vi "Scanner - Top VI.vi"(8 "error in":errorcluster) -> (0 "error out":errorcluster)   [LabVIEW 2024, in "Session Scanner.lvlib"]
uses:
  Session Scanner.lvlib
  Scanner Queue - Dequeue.vi
  User Interface/UI Queue - Enqueue.vi
  Scanner Queue - Enqueue.vi
  Support/General Type Defs/Global Data.vi
  Scanner Queue - Destroy.vi
  User Interface/User Interface.lvlib
  Support/General Type Defs/General Type Defs.lvlib
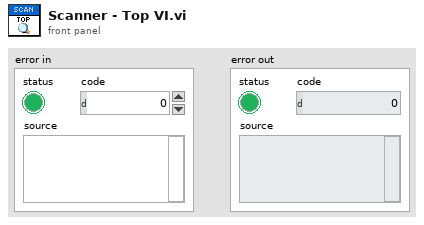
[diagram p1: front panel]
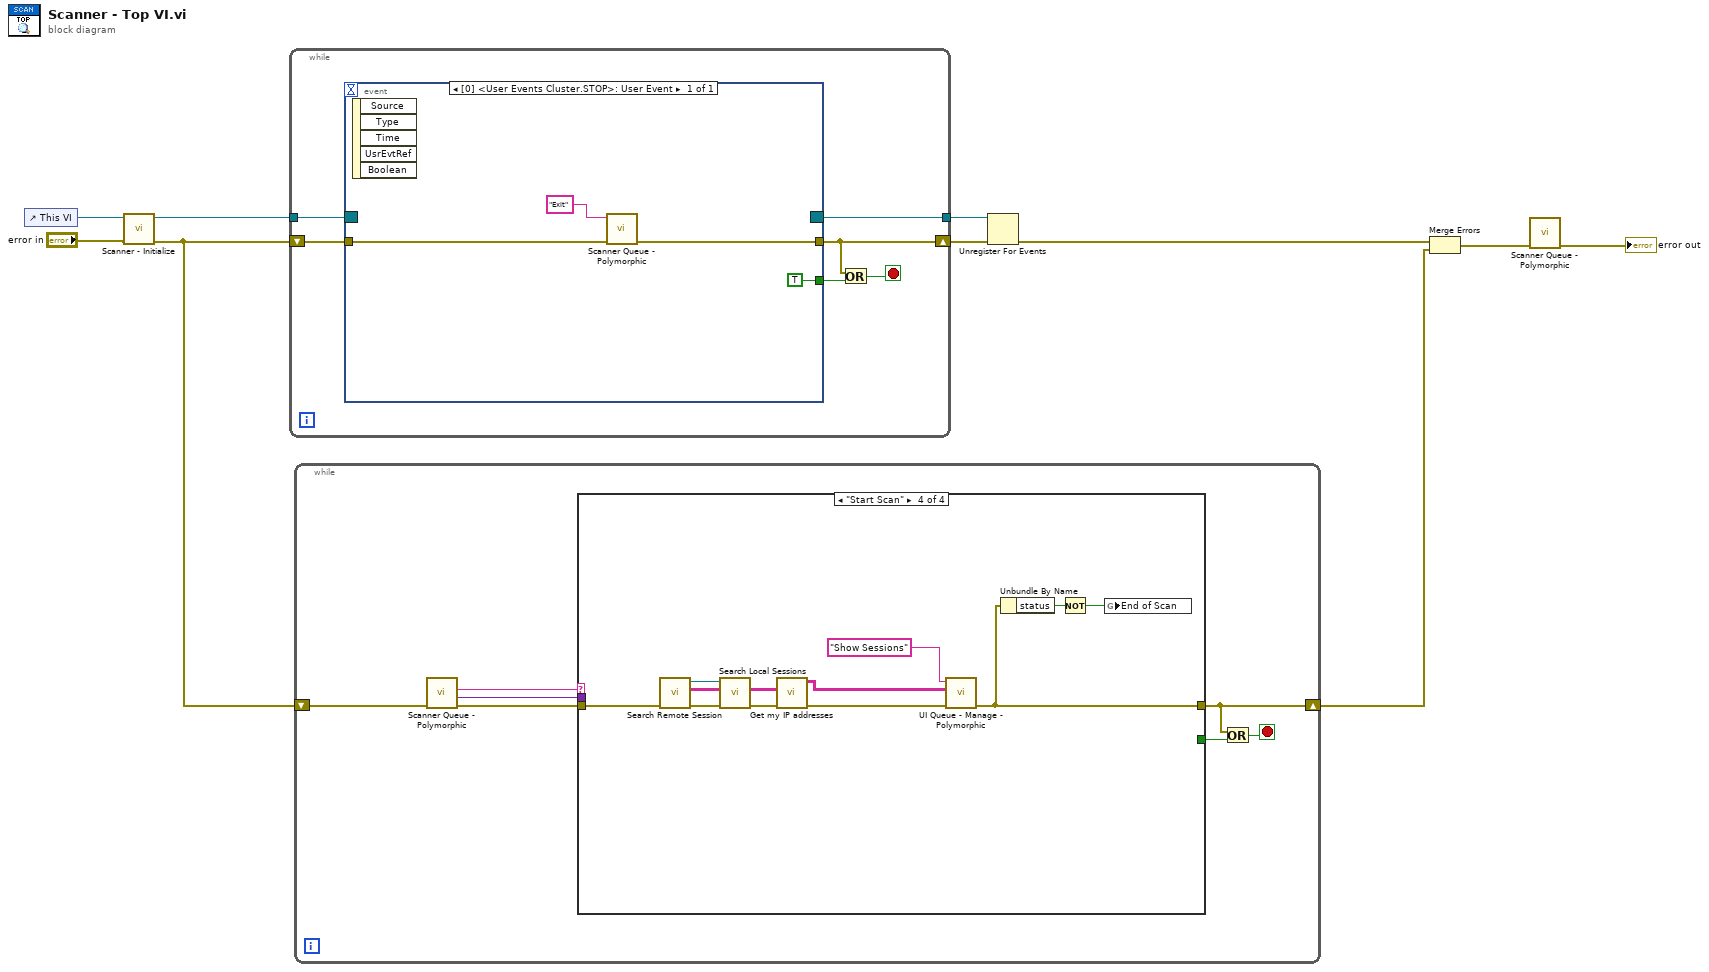
[diagram p0: block diagram]
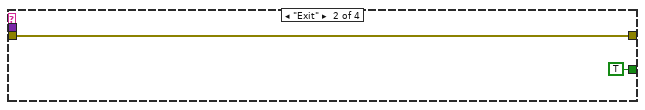
[diagram p3: hidden frame]
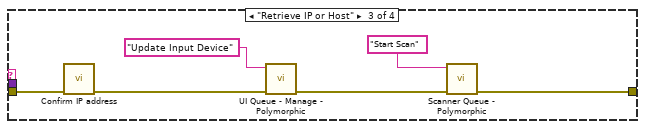
[diagram p4: hidden frame]
diagram:
  n1 = control-ref of="This VI"() -> (w1:refnum<vi>)
  n2 = call "Scanner - Initialize.vi"("error in (no error)"="error in", "VI In"=w1) -> ("error out"=w6:errorcluster, "Event Registration Out"=w9:refnum<event-registration>)  [unwired: 8 in]
  n3 = while {
    tunnel: w9 -> [w16]
    shift-right: [w11] -> w8
    shift-left: w6 -> [w15]
    tunnel: [w14] -> w7
    stop <- w12 stop-if-true
    n4 = event shown="[0] <User Events Cluster.STOP>: User Event" {
      selector: w16 -> [_]
      dyn-events: [_] -> w14
      timeout: _ -> [_]
      tunnel: w15 -> [w19]
      tunnel: [w20] -> w11
      tunnel: [TRUE] -> w13
      event User Event {
        n5 = event-data() -> ()  [unwired: 1 in, 5 out]
        n6 = call-poly "Scanner Queue - Polymorphic.vi"("error in"=w19, "Message"="Exit") -> ("error out"=w20:errorcluster)  [unwired: 9 in]
      }
    }
    n7 = Or(x=w11, y=w13) -> (x .or. y?=w12:bool)
  }
  n8 = while {
    shift-right: [w21] -> w4
    shift-left: w6 -> [w27]
    stop <- w22 stop-if-true
    n9 = call-poly "Scanner Queue - Polymorphic.vi"("error in"=w27) -> ("error out"=w24:errorcluster, "Message Data"=w25:variant, "Message"=w26:string)  [unwired: 8 in]
    n10 = case shown="\"Start Scan\"" w26 {
      tunnel: w25 -> [_ _ _ _]
      tunnel: w24 -> [w28 w29 w36 w48]
      tunnel: [w28 w29 w32 w42] -> w21
      tunnel: [_ TRUE _ _] -> w23
      frame "IDLE", Default {
      }
      frame "Exit" {
      }
      frame "Retrieve IP or Host" {
        n11 = call "Confirm IP address.vi"("error in"=w36) -> ("error out"=w35:errorcluster)  [unwired: 10 in]
        n12 = call-poly "UI Queue - Manage - Polymorphic.vi"("error in"=w35, "Message"="Update Input Device") -> ("error out"=w33:errorcluster)  [unwired: 9 in]
        n13 = call-poly "Scanner Queue - Polymorphic.vi"("error in"=w33, "Message"="Start Scan") -> ("error out"=w32:errorcluster)  [unwired: 9 in]
      }
      frame "Start Scan" {
        n14 = call "Search Remote Session.vi"("error in"=w48) -> ("error out"=w46:errorcluster, "sessions out"=w39:string[][], "SSH session out"=w37:refnum<class "OpenSSH Client.lvclass">)  [unwired: 7 in, 1 out]
        n15 = call "Search Local Sessions.vi"("error in"=w46, "sessions in"=w39, "SSH session in"=w37) -> ("error out"=w45:errorcluster, "sessions out"=w38:string[][])  [unwired: 7 in]
        n16 = call "Get my IP addresses.vi"("error in (no error)"=w45, "Sessions Detected"=w38) -> ("error out"=w44:errorcluster, "Sessions Detected from this PC"=w43:string[][])  [unwired: 8 in]
        n17 = call-poly "UI Queue - Manage - Polymorphic.vi"("error in"=w44, "Value"=w43, "Message"="Show Sessions") -> ("error out"=w42:errorcluster)  [unwired: 8 in]
        n18 = Unbundle By Name(w42) -> ("status"=w41:bool)
        n19 = Not(x=w41) -> (.not. x?=w40:bool)
        n20 = global write "Global Data.vi" "End of Scan"(w40) -> ()
      }
    }
    n21 = Or(x=w21, y=w23) -> (x .or. y?=w22:bool)
  }
  n22 = Unregister For Events(event registration refnum=w7, error in=w8) -> (error out=w5:errorcluster)
  n23 = Merge Errors(w5, w4) -> (w3:errorcluster)
  n24 = call-poly "Scanner Queue - Polymorphic.vi"("error in"=w3) -> ("error out"=→"error out":errorcluster)  [unwired: 10 in]
